vi "Page_Windows_Security_Initialize.vi"(8 "error in (no error)":errorcluster, 9 "ctlReferences":T1, 11 "AB_Application in":refnum<class "AB_Application.lvclass">) -> (0 "error out":errorcluster, 3 "AB_Application out":refnum<class "AB_Application.lvclass">)   [LabVIEW 2020, in "AB_Application.lvclass"]
uses:
  <vilib>/AppBuilder/AB_Classes/Application/AB_Application.lvclass
  <resource>/Framework/Providers/Builds/AppBuilder/AB_UI_Page_Windows_Security_References.ctl
  <resource>/Framework/Providers/Common/provcom_BrowseProjectFile.ctl
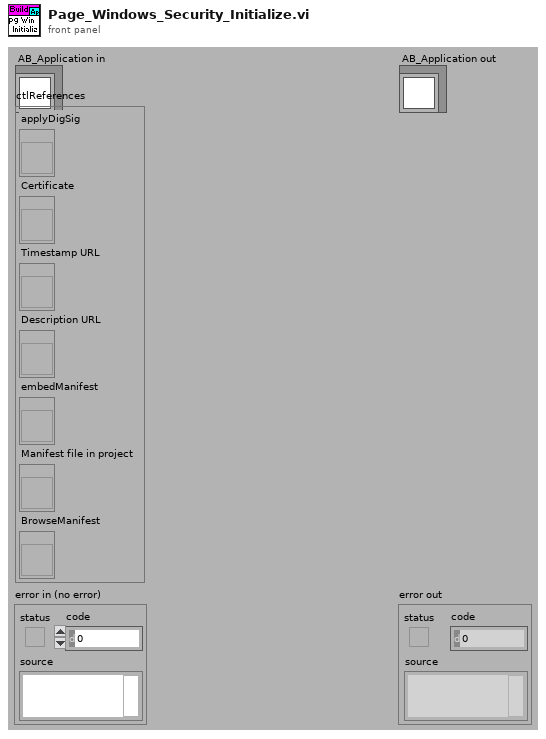
[diagram p1: front panel]
types:
  T1 = typedef "AB_UI_Page_Windows_Security_References.ctl" = cluster{"applyDigSig":refnum<vi>, "Certificate":refnum<vi>, "Timestamp URL":refnum<vi>, "Description URL":refnum<vi>, "embedManifest":refnum<vi>, "Manifest file in project":refnum<vi>, "BrowseManifest":refnum<vi>}
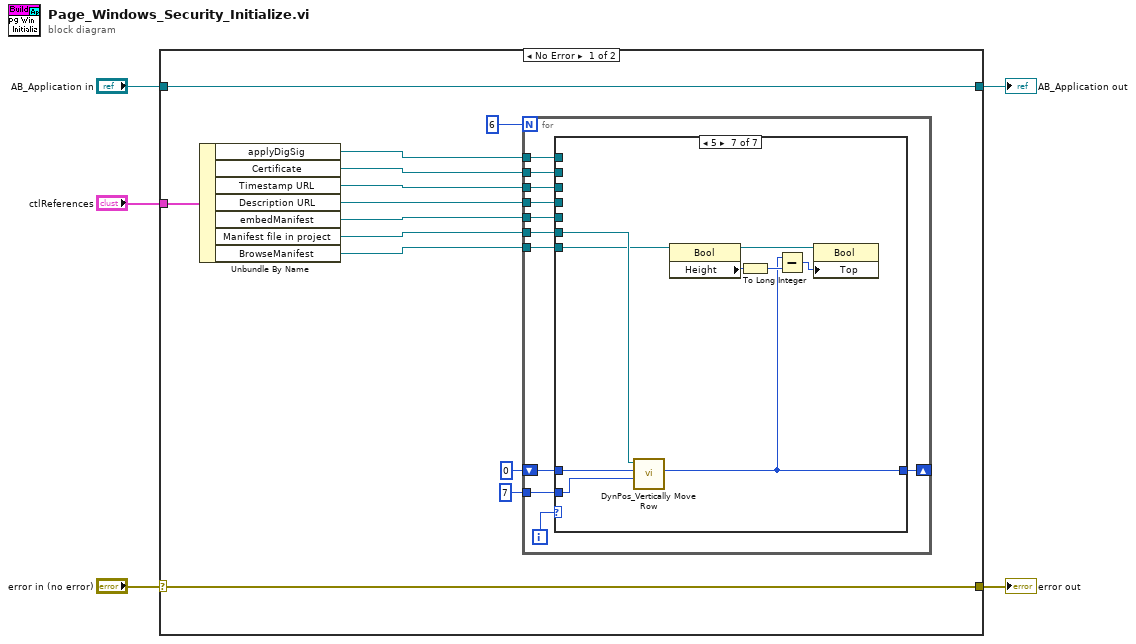
[diagram p0: block diagram]
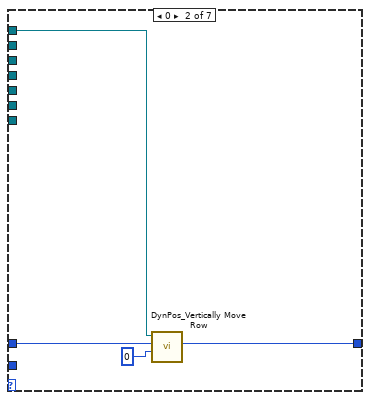
[diagram p3: hidden frame]
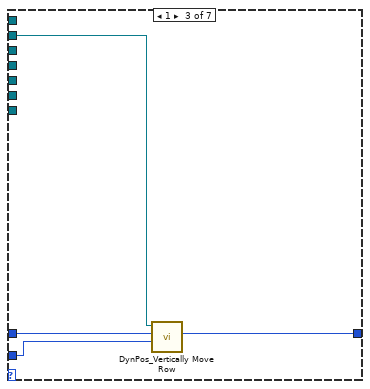
[diagram p4: hidden frame]
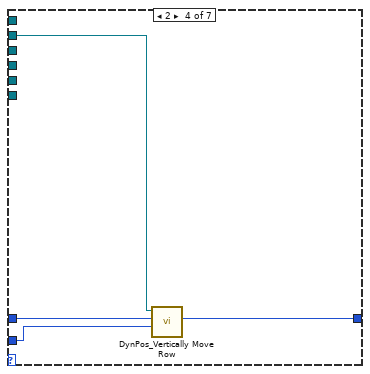
[diagram p5: hidden frame]
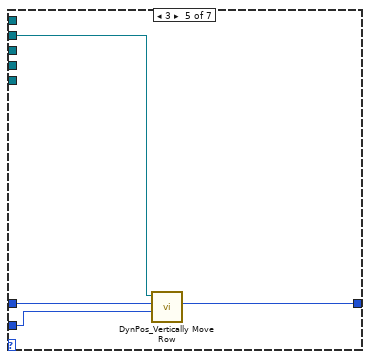
[diagram p6: hidden frame]
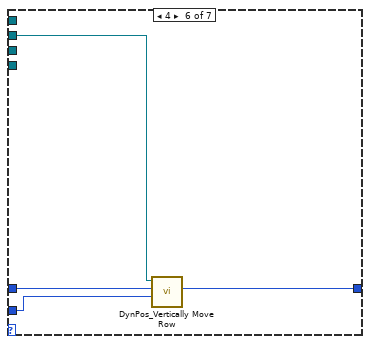
[diagram p7: hidden frame]
diagram:
  n1 = case shown="No Error" "error in (no error)" {
    selector: "error in (no error)" -> [w18 w61]
    tunnel: [w18 w61] -> w4
    tunnel: [w17 w60] -> w2
    tunnel: "AB_Application in" -> [w17 w60]
    tunnel: "ctlReferences" -> [w16 _]
    frame No Error {
      n2 = Unbundle By Name(w16) -> ("applyDigSig"=w14:refnum<vi>, "Certificate"=w11:refnum<vi>, "Timestamp URL"=w10:refnum<vi>, "Description URL"=w9:refnum<vi>, "embedManifest"=w8:refnum<vi>, "Manifest file in project"=w7:refnum<vi>, "BrowseManifest"=w6:refnum<vi>)
      n3 = for {
        N: 6 -> [_]
        tunnel: w14 -> [w29]
        shift-right: [w26] -> _
        shift-left: 0 -> [w27]
        tunnel: 7 ("Bottom of last control") -> [w25]
        tunnel: w11 -> [w24]
        tunnel: w10 -> [w23]
        tunnel: w9 -> [w22]
        tunnel: w8 -> [w21]
        tunnel: w7 -> [w20]
        tunnel: w6 -> [w19]
        i -> [w28]
        n4 = case shown="5" w28 {
          tunnel: w29 -> [_ w33 _ _ _ _ _]
          tunnel: w27 -> [w30 w32 w38 w42 w46 w50 w59]
          tunnel: [w30 w31 w37 w41 w45 w49 w52] -> w26
          tunnel: w25 -> [_ _ w36 w40 w44 w48 w58]
          tunnel: w24 -> [_ _ w35 _ _ _ _]
          tunnel: w23 -> [_ _ _ w39 _ _ _]
          tunnel: w22 -> [_ _ _ _ w43 _ _]
          tunnel: w21 -> [_ _ _ _ _ w47 _]
          tunnel: w20 -> [_ _ _ _ _ _ w57]
          tunnel: w19 -> [_ _ _ _ _ _ w51]
          frame Default {
          }
          frame 0 {
            n5 = call <vilib>:"DynPos_Vertically Move Row.vi"("Pixel separation (6)"=0, "Bottom of last control"=w32, "Control"=w33) -> ("Bottom pixel"=w31:i32)  [unwired: 1 in, 7 out]
          }
          frame 1 {
            n6 = call <vilib>:"DynPos_Vertically Move Row.vi"("Pixel separation (6)"=w36, "Bottom of last control"=w38, "Control"=w35) -> ("Bottom pixel"=w37:i32)  [unwired: 1 in, 7 out]
          }
          frame 2 {
            n7 = call <vilib>:"DynPos_Vertically Move Row.vi"("Pixel separation (6)"=w40, "Bottom of last control"=w42, "Control"=w39) -> ("Bottom pixel"=w41:i32)  [unwired: 1 in, 7 out]
          }
          frame 3 {
            n8 = call <vilib>:"DynPos_Vertically Move Row.vi"("Pixel separation (6)"=w44, "Bottom of last control"=w46, "Control"=w43) -> ("Bottom pixel"=w45:i32)  [unwired: 1 in, 7 out]
          }
          frame 4 {
            n9 = call <vilib>:"DynPos_Vertically Move Row.vi"("Pixel separation (6)"=w48, "Bottom of last control"=w50, "Control"=w47) -> ("Bottom pixel"=w49:i32)  [unwired: 1 in, 7 out]
          }
          frame 5 {
            n10 = call <vilib>:"DynPos_Vertically Move Row.vi"("Pixel separation (6)"=w58, "Bottom of last control"=w59, "Control"=w57) -> ("Bottom pixel"=w52:i32)  [unwired: 1 in, 7 out]
            n11 = property class="Bool"(reference=w51) -> (reference out=w53:refnum<vi>, "Height"=w54:u32)  [unwired: 1 in, 1 out]
            n12 = To Long Integer(number=w54) -> (32bit integer=w56:i32)
            n13 = Subtract(x=w52, y=w56) -> (x-y=w55:i32)
            n14 = property class="Bool"(reference=w53, "Top"=w55) -> ()  [unwired: 1 in, 2 out]
          }
        }
      }
    }
    frame Error {
    }
  }
  "error out" <- w4
  "AB_Application out" <- w2
